vi "LF_maker.vi"() -> ()   [LabVIEW 2014]
uses:
  <vilib>/Utility/file.llb/Read From Spreadsheet File (string).vi
  <vilib>/Utility/file.llb/Read From Spreadsheet File (I64).vi
  <vilib>/Utility/file.llb/Read From Spreadsheet File (DBL).vi
  <vilib>/Utility/file.llb/Write To Spreadsheet File (DBL).vi
panel:
  in  "피험자이름":path=path "C:/Users/Jaehong/Desktop/Classifiers/HRV_EEG/ERP_total/강병훈/ERP_total.txt"
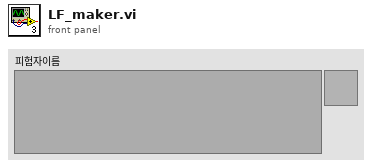
[diagram p1: front panel]
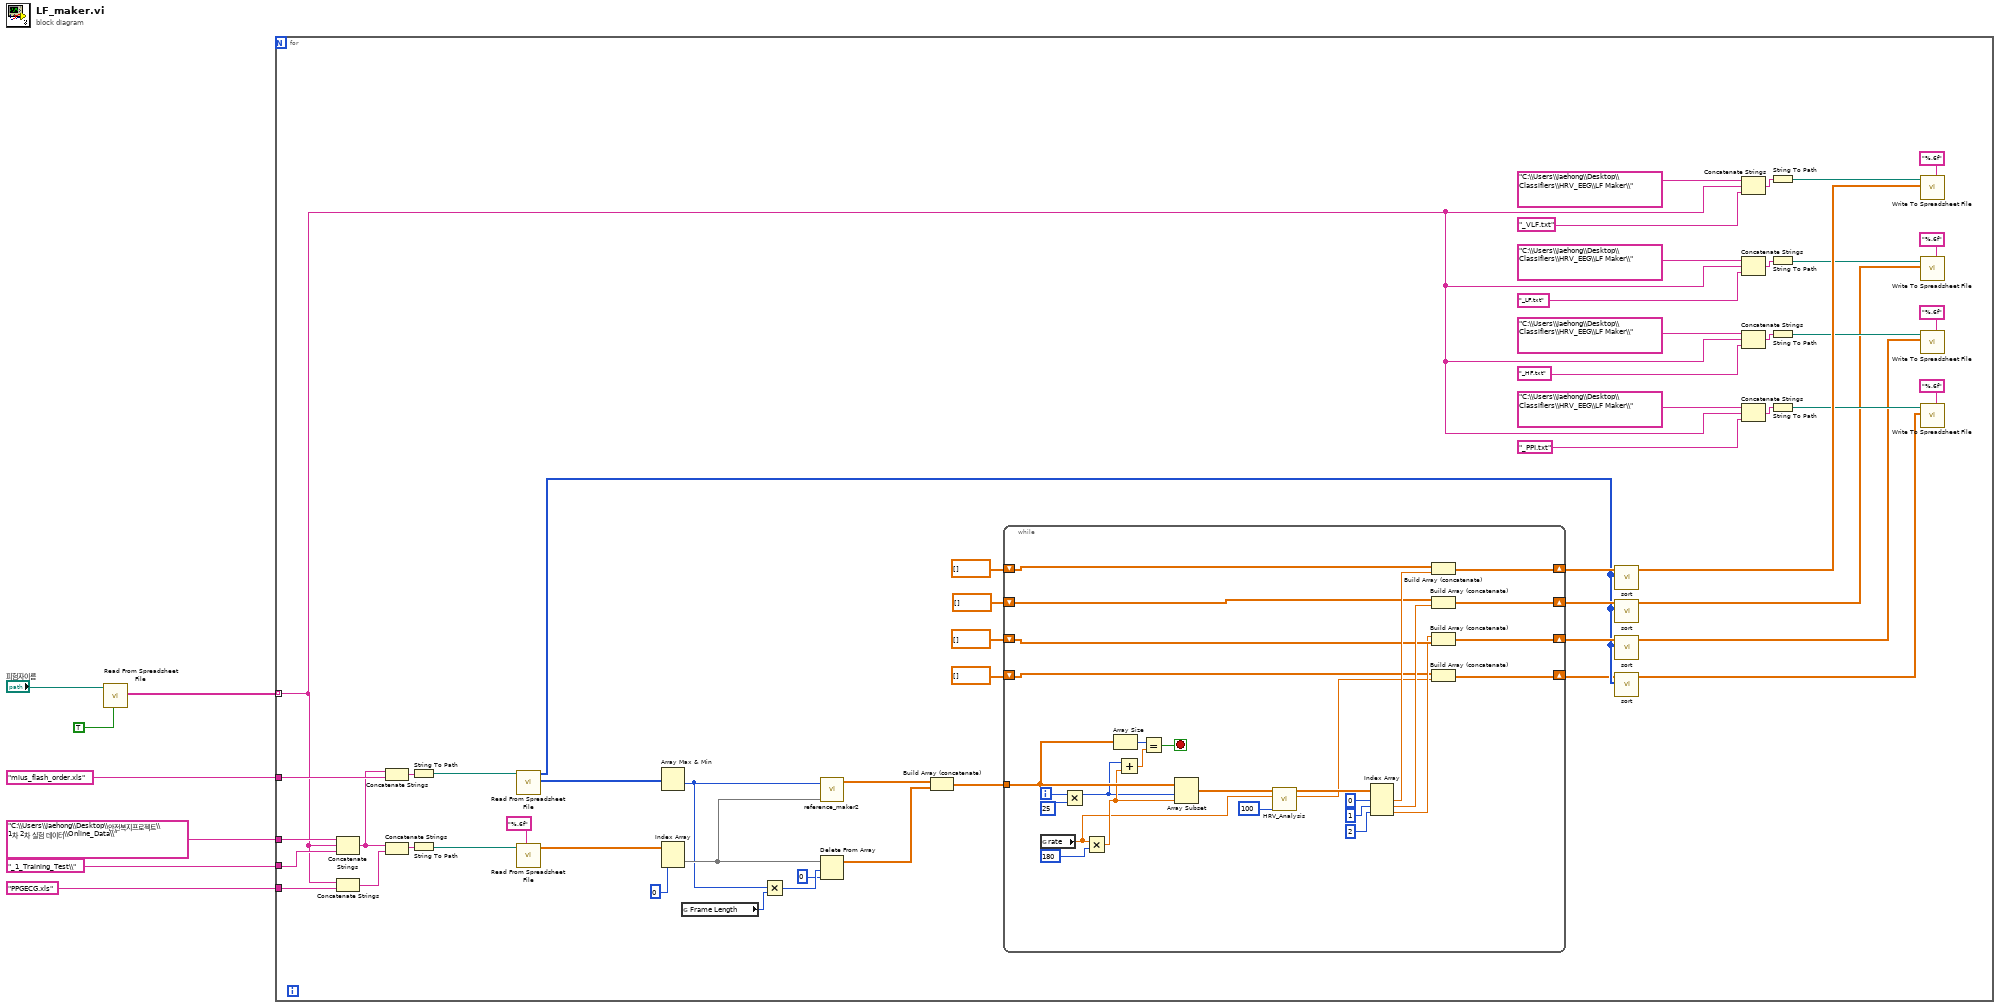
[diagram p0: block diagram]
diagram:
  n1 = call-poly <vilib>:"Read From Spreadsheet File.vi"("transpose (no:F)"=TRUE, "file path (dialog if empty)"="피험자이름") -> ("first row"=w5:string[])  [unwired: 5 in, 4 out]
  n2 = for {
    tunnel: w5 -> [w17] mode=indexing
    tunnel: "C:\\Users\\Jaehong\\Desktop\\안전복지프로젝트\\1차 2차 실험 데이터\\Online_Data\\" -> [w59]
    tunnel: "_1_Training_Test\\" -> [w58]
    tunnel: "PPGECG.xls" -> [w57]
    tunnel: "mius_flash_order.xls" -> [w54]
    n3 = Concatenate Strings(w59, w17, w58) -> (w52:string)
    n4 = Concatenate Strings(w17, w57) -> (w56:string)
    n5 = Concatenate Strings(w52, w54) -> (w53:string)
    n6 = Concatenate Strings(w52, w56) -> (w55:string)
    n7 = String To Path(string=w53) -> (path=w51:path)
    n8 = String To Path(string=w55) -> (path=w60:path)
    n9 = call-poly <vilib>:"Read From Spreadsheet File.vi"("file path (dialog if empty)"=w51) -> ("first row"=w34:i64[], "all rows"=w29:i64[][])  [unwired: 6 in, 3 out]
    n10 = call-poly <vilib>:"Read From Spreadsheet File.vi"("format (%.3f)"="%.6f", "file path (dialog if empty)"=w60) -> ("all rows"=w62:dbl[][])  [unwired: 5 in, 4 out]
    n11 = Array Max & Min(array=w34) -> (min value=w33:i64)  [unwired: 3 out]
    n12 = Index Array(array=w62, index (col)=0 ("index")) -> (element=w50:dbl[])  [unwired: 1 in]
    n13 = global read "Control_Panel.vi" "Frame Length"() -> (w49:i32)
    n14 = Multiply(x=w33, y=w49) -> (x*y=w48:i64)
    n15 = call "reference_maker2.vi"("Raw_PPG"=w50, "start_index"=w33) -> ("reference"=w46:dbl[])  [unwired: 9 in]
    n16 = Delete From Array(array=w50, length=w48, index=0) -> (array with subset deleted=w45:dbl[])  [unwired: 1 out]
    n17 = Build Array (concatenate)(w46, w45) -> (w44:dbl[])
    n18 = while {
      tunnel: w44 -> [w90]
      shift-right: [w79] -> w32
      shift-left: dbl[] [] -> [w78]
      shift-right: [w74] -> w31
      shift-left: dbl[] [] -> [w73]
      shift-right: [w71] -> w30
      shift-left: dbl[] [] -> [w70]
      shift-right: [w68] -> w28
      shift-left: dbl[] [] -> [w66]
      i -> [w89]
      stop <- w85 stop-if-true
      n19 = global read "Control_Panel.vi" "rate"() -> (w83:dbl)
      n20 = Multiply(x=w89, y=25) -> (x*y=w65:i32)
      n21 = Multiply(x=w83, y=180) -> (x*y=w88:dbl)
      n22 = Array Size(array=w90) -> (size(s)=w87:i32)
      n23 = Add(x=w65, y=w88) -> (x+y=w86:dbl)
      n24 = Equal?(x=w87, y=w86) -> (x = y?=w85:bool)
      n25 = Array Subset(array=w90, index=w65, length=w88) -> (w84:dbl[])
      n26 = call "HRV_Analysis.vi"("Frame Length"=100, "Sample Rate"=w83, "PPG_Data"=w84) -> ("PPI"=w67:dbl, "PRV% (VLF, LF, HF)"=w81:dbl[])  [unwired: 7 in]
      n27 = Index Array(array=w81, index #1=0 ("index"), index #2=1 ("index"), index #3=2 ("index")) -> (element #1=w80:dbl, element #2=w72:dbl, element #3=w69:dbl)
      n28 = Build Array (concatenate)(w78, w80) -> (w79:dbl[])
      n29 = Build Array (concatenate)(w73, w72) -> (w74:dbl[])
      n30 = Build Array (concatenate)(w69, w70) -> (w71:dbl[])
      n31 = Build Array (concatenate)(w66, w67) -> (w68:dbl[])
    }
    n32 = call "sort.vi"("mius_flash_order"=w29, "HRV_data"=w32) -> ("appended array"=w27:dbl[][])  [unwired: 9 in]
    n33 = call "sort.vi"("mius_flash_order"=w29, "HRV_data"=w31) -> ("appended array"=w8:dbl[][])  [unwired: 9 in]
    n34 = call "sort.vi"("mius_flash_order"=w29, "HRV_data"=w30) -> ("appended array"=w9:dbl[][])  [unwired: 9 in]
    n35 = call "sort.vi"("mius_flash_order"=w29, "HRV_data"=w28) -> ("appended array"=w10:dbl[][])  [unwired: 9 in]
    n36 = Concatenate Strings("C:\\Users\\Jaehong\\Desktop\\Classifiers\\HRV_EEG\\LF Maker\\", w17, "_VLF.txt") -> (w36:string)
    n37 = Concatenate Strings("C:\\Users\\Jaehong\\Desktop\\Classifiers\\HRV_EEG\\LF Maker\\", w17, "_LF.txt") -> (w25:string)
    n38 = Concatenate Strings("C:\\Users\\Jaehong\\Desktop\\Classifiers\\HRV_EEG\\LF Maker\\", w17, "_HF.txt") -> (w22:string)
    n39 = Concatenate Strings("C:\\Users\\Jaehong\\Desktop\\Classifiers\\HRV_EEG\\LF Maker\\", w17, "_PPI.txt") -> (w19:string)
    n40 = String To Path(string=w36) -> (path=w39:path)
    n41 = String To Path(string=w25) -> (path=w15:path)
    n42 = String To Path(string=w22) -> (path=w13:path)
    n43 = String To Path(string=w19) -> (path=w11:path)
    n44 = call-poly <vilib>:"Write To Spreadsheet File.vi"("format (%.3f)"="%.6f", "2D data"=w27, "file path (dialog if empty)"=w39) -> ()  [unwired: 5 in, 1 out]
    n45 = call-poly <vilib>:"Write To Spreadsheet File.vi"("format (%.3f)"="%.6f", "2D data"=w8, "file path (dialog if empty)"=w15) -> ()  [unwired: 5 in, 1 out]
    n46 = call-poly <vilib>:"Write To Spreadsheet File.vi"("format (%.3f)"="%.6f", "2D data"=w9, "file path (dialog if empty)"=w13) -> ()  [unwired: 5 in, 1 out]
    n47 = call-poly <vilib>:"Write To Spreadsheet File.vi"("format (%.3f)"="%.6f", "2D data"=w10, "file path (dialog if empty)"=w11) -> ()  [unwired: 5 in, 1 out]
  }
